vi "Assembly Line Image Generator.vi"(9 "assembly line input":T1, 10 "how many":i32=50, 11 "Queue in":refnum<queue>) -> (0 "error out":errorcluster)   [LabVIEW 2023]
doc: "Given an image for a correct board, generate the requested number of randomly correct or incorrect image (with approximately 75% success rate) and add them to the queue."
uses:
  Assembly Line Input.ctl
  Board Image.ctl
  Board Type Enum.ctl
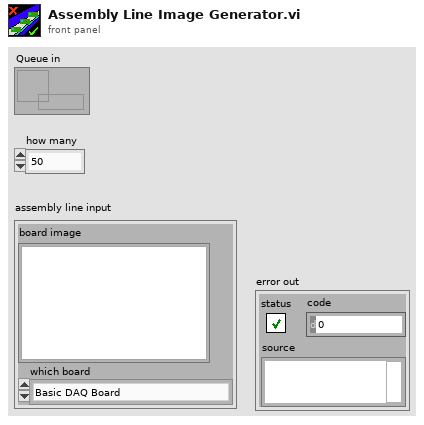
[diagram p1: front panel]
types:
  T1 = typedef "Assembly Line Input.ctl" = cluster{"board image":T2, "which board":T3}
  T2 = typedef "Board Image.ctl" = picture
  T3 = typedef "Board Type Enum.ctl" = enum16{"Basic DAQ Board", "Elite DAQ Board", "GPIB Board"}
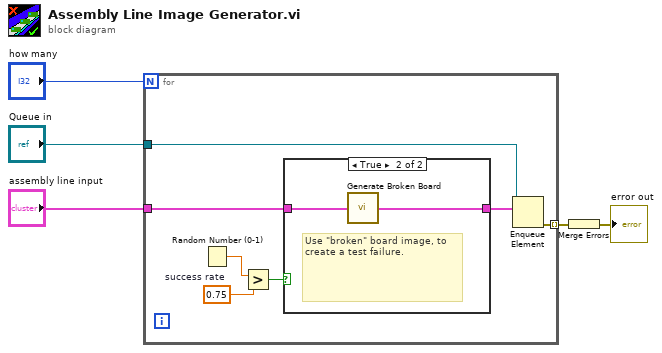
[diagram p0: block diagram]
diagram:
  n1 = for {
    N: "how many" -> [_]
    tunnel: "Queue in" -> [w12]
    tunnel: "assembly line input" -> [w8]
    tunnel: [w6] -> w2 mode=indexing
    w10 = 0.75  # success rate
    n2 = Random Number (0-1)() -> (number: 0 to 1=w11:dbl)
    n3 = Greater?(x=w11, y=w10) -> (0:w9:bool)
    n4 = case shown="True" w9 {
      tunnel: w8 -> [w13 w15]
      tunnel: [w13 w14] -> w7
      frame False {
        # "Use \"correct\" image from input."
      }
      frame True {
        # "Use \"broken\" board image, to create a test failure."
        n5 = call "Generate Broken Board.vi"("Assembly Line Input"=w15) -> ("Assembly Line Input out"=w14:T1)
      }
    }
    n6 = Enqueue Element(queue=w12, element=w7) -> (error out=w6:errorcluster)  [unwired: 2 in, 2 out]
  }
  n7 = Merge Errors(w2) -> (→"error out":errorcluster)
